vi "error_analysis.vi"(8 "tLength":i32, 9 "t0":i32, 11 "data in (um)":dbl[](array[numeric])) -> (0 "rms (one) (um)":dbl, 1 "max err (um)":dbl, 2 "rms (all) (um)":dbl, 3 "data out (um)":dbl[](array[numeric]))   [LabVIEW 2019]
uses:
  <vilib>/Analysis/5stat.llb/RMS (DBL).vi
  <vilib>/Analysis/NI_AALPro.lvlib
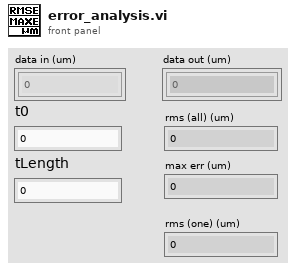
[diagram p1: front panel]
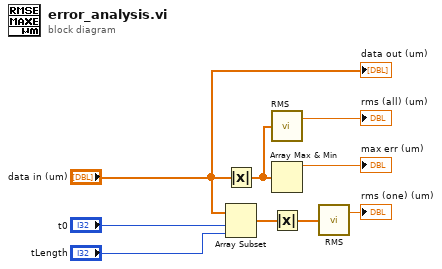
[diagram p0: block diagram]
diagram:
  n1 = Absolute Value(x="data in (um)") -> (abs(x)=w6:dbl[])
  n2 = Array Subset(array="data in (um)", index="t0", length="tLength") -> (w5:dbl[])
  n3 = call-poly <vilib>:"RMS.vi"("X"=w6) -> ("rms value"=→"rms (all) (um)":dbl)  [unwired: 1 out]
  n4 = Array Max & Min(array=w6) -> (max value=→"max err (um)":dbl)  [unwired: 3 out]
  n5 = Absolute Value(x=w5) -> (abs(x)=w4:dbl[])
  n6 = call-poly <vilib>:"RMS.vi"("X"=w4) -> ("rms value"=→"rms (one) (um)":dbl)  [unwired: 1 out]
  "data out (um)" <- "data in (um)"
